vi "Exec TA Binding.vi"(8 "error in (no error)":errorcluster, 10 "Array of States LUT":variant[](array[variant]), 11 "Motions in":refnum<class "Motions.lvclass">) -> (0 "error out":errorcluster, 3 "Motions out":refnum<class "Motions.lvclass">)   [LabVIEW 2016, in "Hardware.lvlib" / "Motions.lvlib" / "Motions.lvclass"]
uses:
  <userlib>/Common Components/Hardware/Abstract System/Motions/Motions/Motions.lvclass
  <userlib>/Common Components/Hardware/Abstract System/Motions/Motions/Motions.lvclass/Motions.ctl
  <vilib>/Utility/error.llb/Error Cluster From Error Code.vi
  <vilib>/ErrorRing/Error Ring.xnode
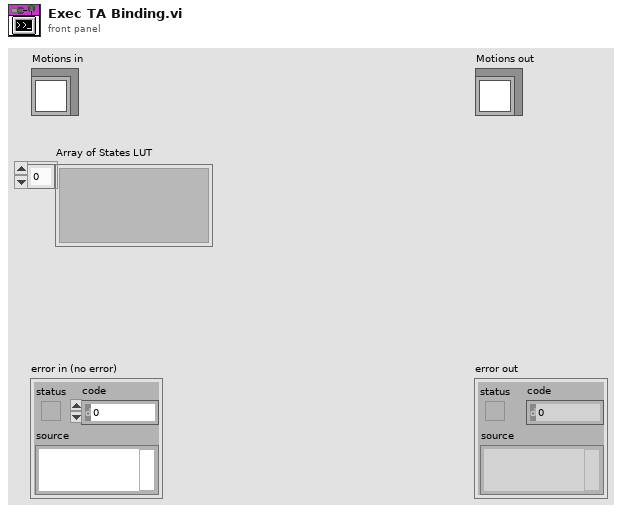
[diagram p1: front panel]
types:
  T1 = typedef "Hardware.lvlib/Motions.lvlib/Motions.lvclass/TA Binding Data.ctl" = cluster{"Triggers":cluster{"Triggers for Array AND":cluster{"Index":u8, "State Name":string}[]}[], "Actions":cluster{"Action Name":string, "Action Data":string}[]}
  T2 = cluster{"Triggers for Array AND":cluster{"Index":u8, "State Name":string}[]}[]
  T3 = cluster{"Action Name":string, "Action Data":string}[]
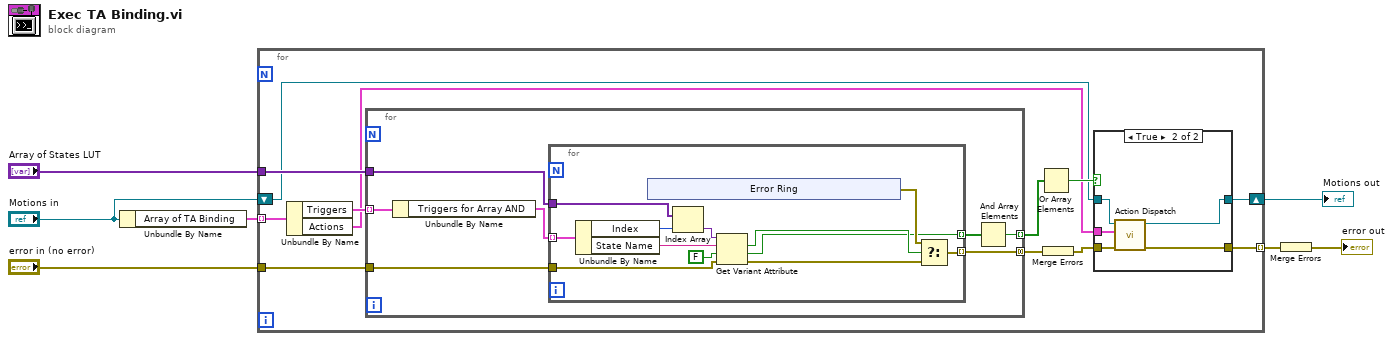
[diagram p0: block diagram]
diagram:
  n1 = Unbundle By Name("Motions in") -> ("Array of TA Binding"=w7:T1[])
  n2 = for {
    tunnel: w7 -> [w19] mode=indexing
    tunnel: "Array of States LUT" -> [w17]
    tunnel: "error in (no error)" -> [w15]
    tunnel: [w8] -> w5 mode=indexing
    shift-right: [w11] -> w1
    shift-left: "Motions in" -> [w12]
    n3 = Unbundle By Name(w19) -> ("Triggers"=w18:T2, "Actions"=w10:T3)
    n4 = for {
      tunnel: w18 -> [w33] mode=indexing
      tunnel: w17 -> [w31]
      tunnel: [w29] -> w16 mode=indexing
      tunnel: w15 -> [w28]
      tunnel: [w27] -> w14 mode=concatenating
      n5 = Unbundle By Name(w33) -> ("Triggers for Array AND"=w32:cluster{"Index":u8, "State Name":string}[])
      n6 = for {
        tunnel: w32 -> [w45] mode=indexing
        tunnel: w31 -> [w44]
        tunnel: [w36] -> w27 mode=indexing
        tunnel: [w35] -> w30 mode=indexing
        tunnel: w28 -> [w34]
        n7 = Unbundle By Name(w45) -> ("Index"=w43:u8, "State Name"=w37:string)
        n8 = xnode "Error Ring"() -> ("error out"=w40:errorcluster)
        n9 = Index Array(array=w44, index=w43) -> (element=w38:variant)
        n10 = Get Variant Attribute(Variant=w38, name=w37, default value (empty Variant)=FALSE, error in=w34) -> (found=w41:bool, value=w35:bool, error out=w39:errorcluster)  [unwired: 1 out]
        n11 = Select(t=w40, s=w41, f=w39) -> (s? t:f=w36:errorcluster)
      }
      n12 = And Array Elements(Boolean array=w30) -> (logical AND=w29:bool)
    }
    n13 = Or Array Elements(Boolean array=w16) -> (logical OR=w13:bool)
    n14 = Merge Errors(w14) -> (w9:errorcluster)
    n15 = case shown="True" w13 {
      tunnel: w12 -> [w21 w26]
      tunnel: [w21 w25] -> w11
      tunnel: w10 -> [_ w24]
      tunnel: w9 -> [w20 w23]
      tunnel: [w20 w22] -> w8
      frame False {
      }
      frame True {
        n16 = call <userlib>:"Action Dispatch.vi"("error in (no error)"=w23, "Actions"=w24, "Motions in"=w26) -> ("error out"=w22:errorcluster, "Motions out"=w25:refnum<class "Motions.lvclass">)  [unwired: 7 in]
      }
    }
  }
  "Motions out" <- w1
  n17 = Merge Errors(w5) -> (→"error out":errorcluster)
